vi "SimpleGit_Item_OnUpdateCommand.vi"(10 "Menu Item In":T1={"Menu Name"="", "Description"="", "Icon File Name"=path "", "Menu Tag"="", "Enabled"=TRUE, "Checked"=FALSE, "Separator"=FALSE, "Batchable"=TRUE, "Weight"=0, "Batch Mode (Ignored if Not Batchable)"=enum."Show If All Items Support Command", "Menu Location"=enum."<None>", "Exclude From Getting Started Window Menu"=FALSE}, 11 "Object":T2) -> (3 "Menu Item Out":T1={"Menu Name"="", "Description"="", "Icon File Name"=path "", "Menu Tag"="", "Enabled"=TRUE, "Checked"=FALSE, "Separator"=FALSE, "Batchable"=TRUE, "Weight"=0, "Batch Mode (Ignored if Not Batchable)"=enum."Show If All Items Support Command", "Menu Location"=enum."<None>", "Exclude From Getting Started Window Menu"=FALSE})   [LabVIEW 2017]
uses:
  <resource>/Framework/Providers/API/ItemRef.ctl
  <resource>/Framework/Providers/API/mxLvMenuItem.ctl
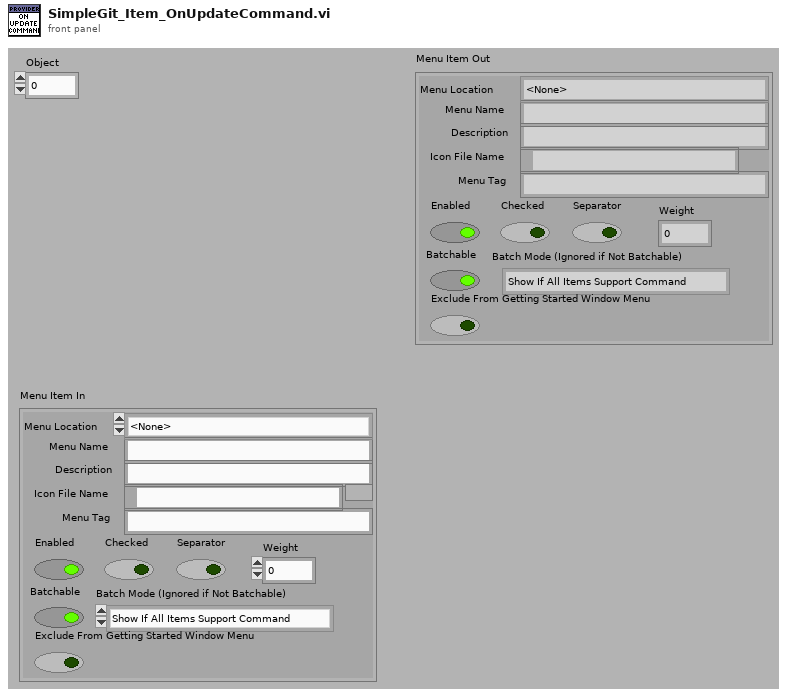
[diagram p1: front panel]
types:
  T1 = typedef "mxLvMenuItem.ctl" = cluster{"Menu Name":string, "Description":string, "Icon File Name":path, "Menu Tag":string, "Enabled":bool, "Checked":bool, "Separator":bool, "Batchable":bool, "Weight":i32, "Batch Mode (Ignored if Not Batchable)":enum32{"Show If All Items Support Command", "Show If Any Items Support Command"}, "Menu Location":enum32{"<None>", "Project", "Project / Build Specifications", "Tools", "Tools / Source Control", "Tools / Real-Time Module", "Help"}, "Exclude From Getting Started Window Menu":bool}
  T2 = typedef "ItemRef.ctl" = u64
  T3 = cluster{"current branch":string, "current commit":string, "Commit Info":string}
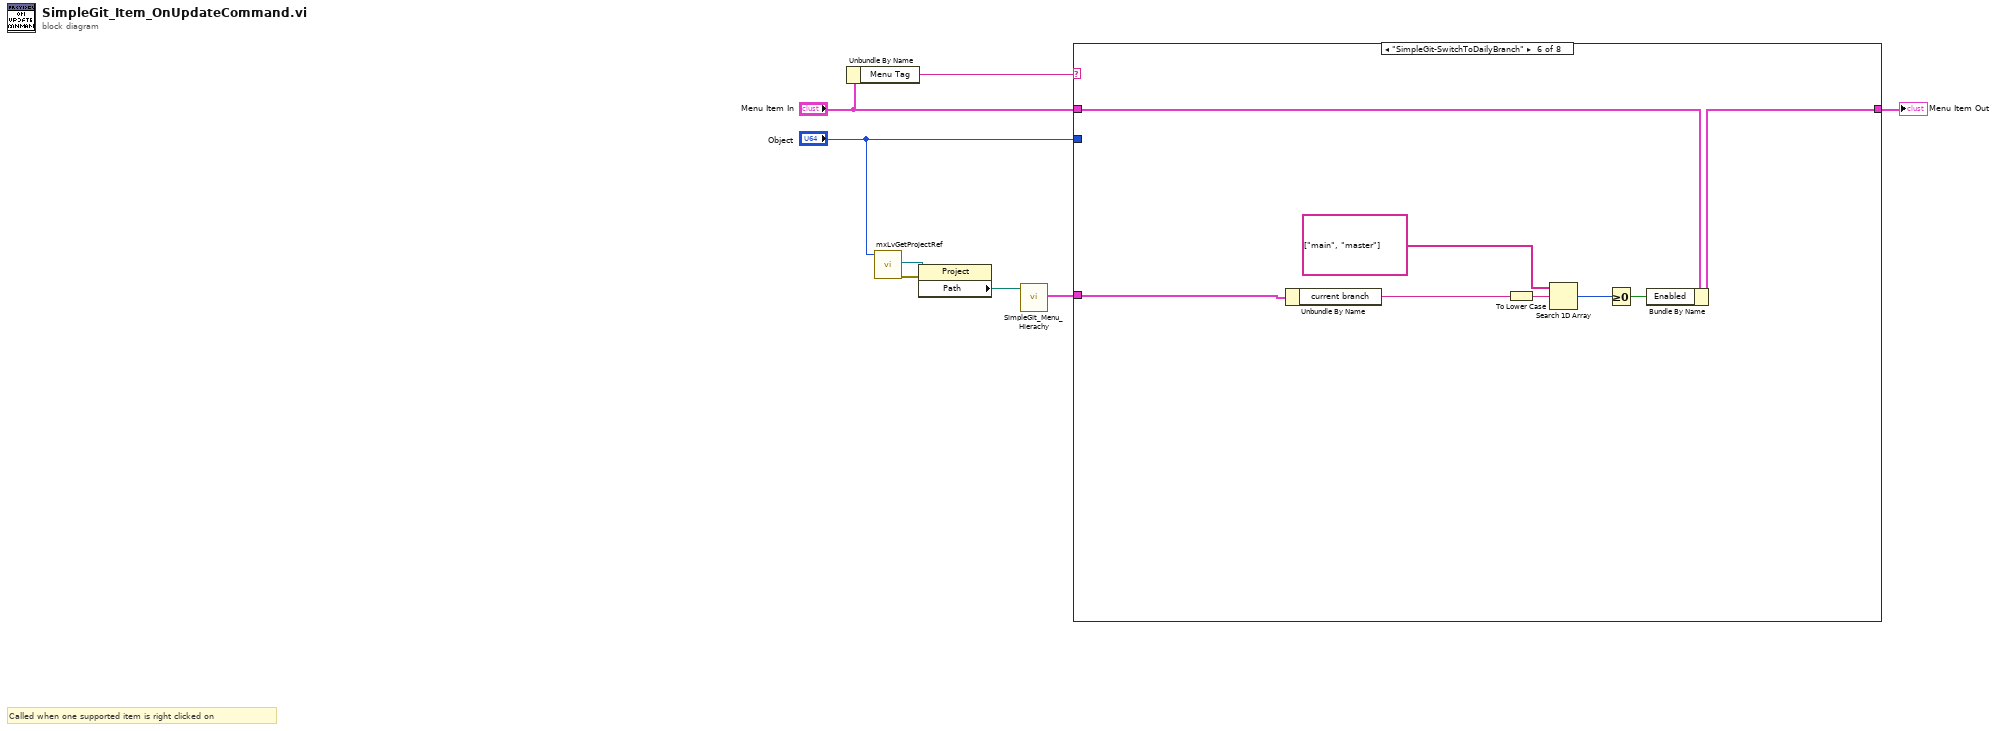
[diagram p0: block diagram]
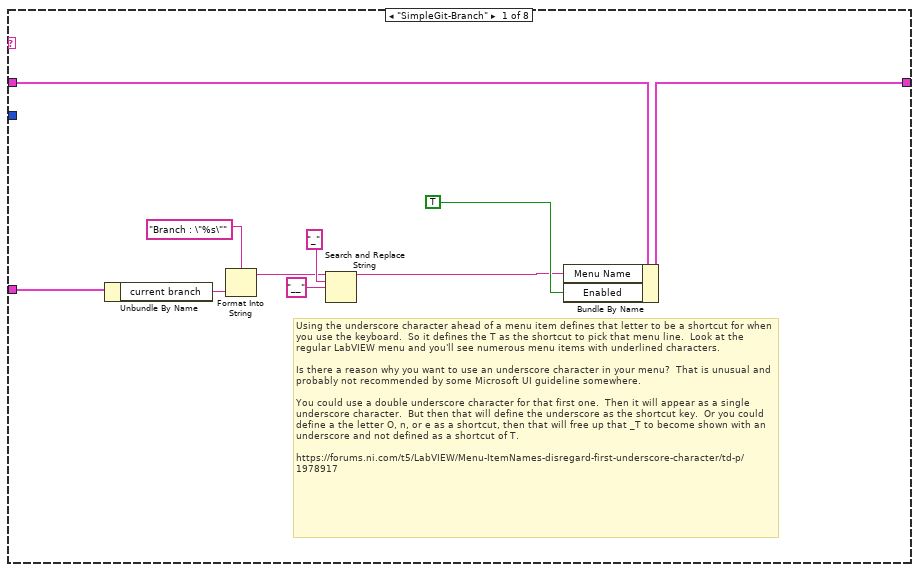
[diagram p2: hidden frame]
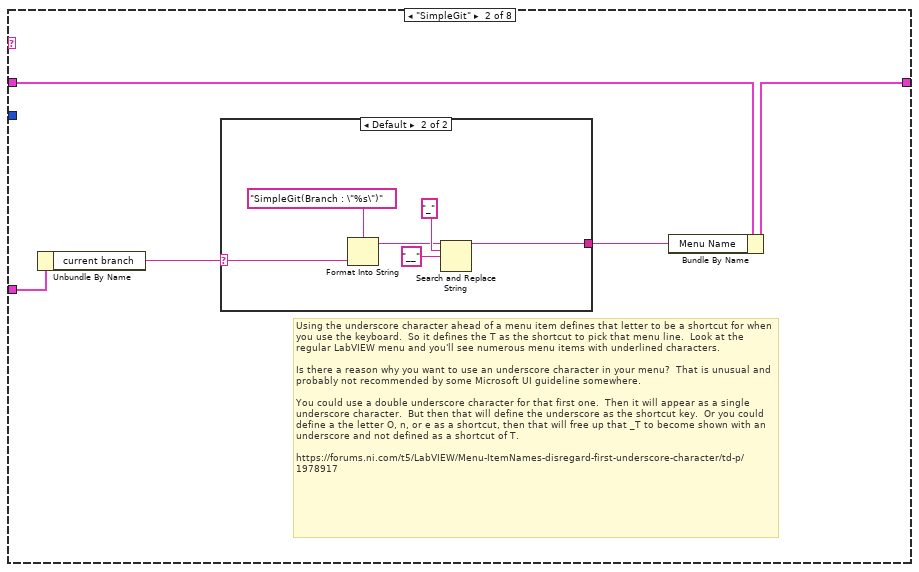
[diagram p3: hidden frame]
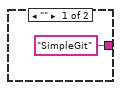
[diagram p4: hidden frame]
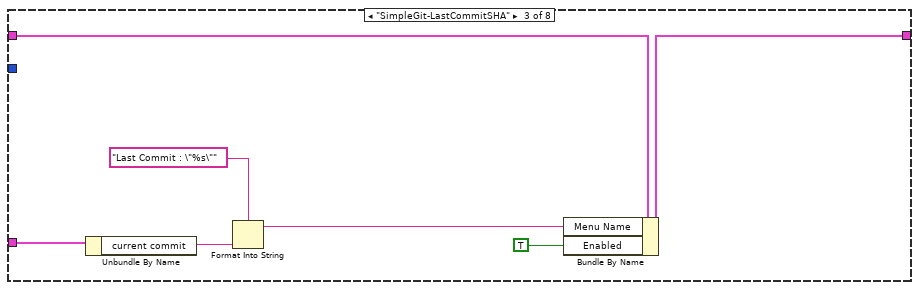
[diagram p5: hidden frame]
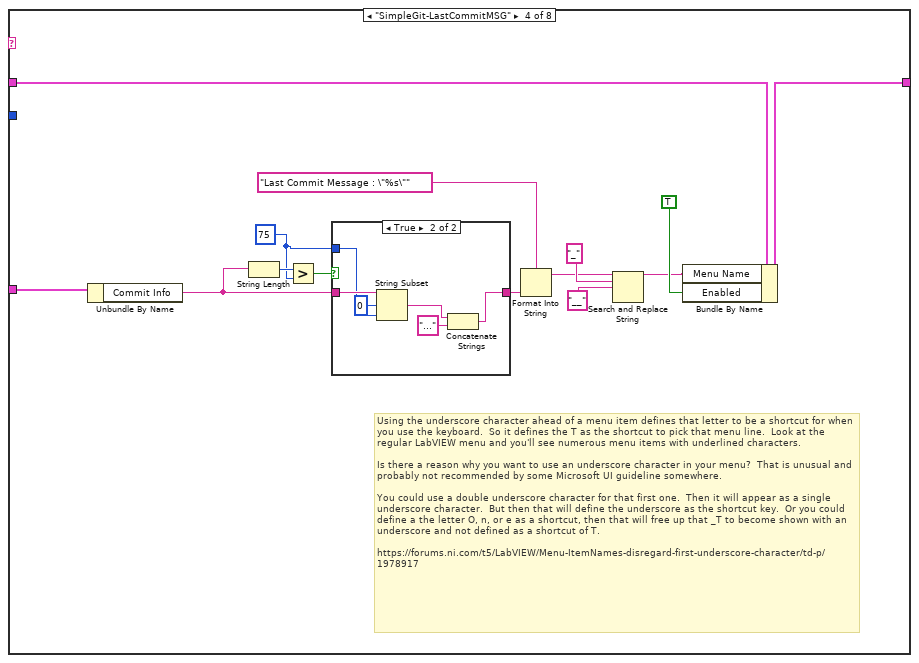
[diagram p6: hidden frame]
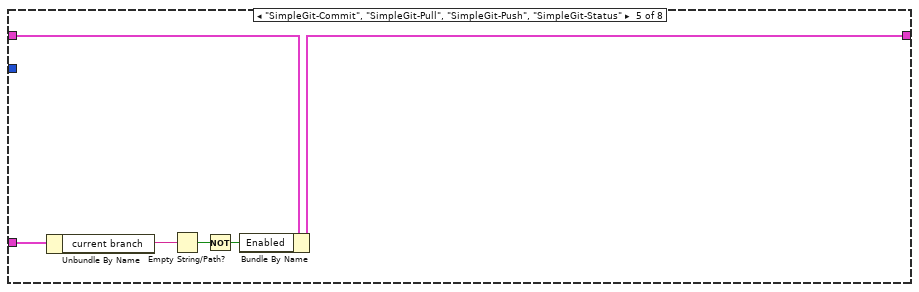
[diagram p8: hidden frame]
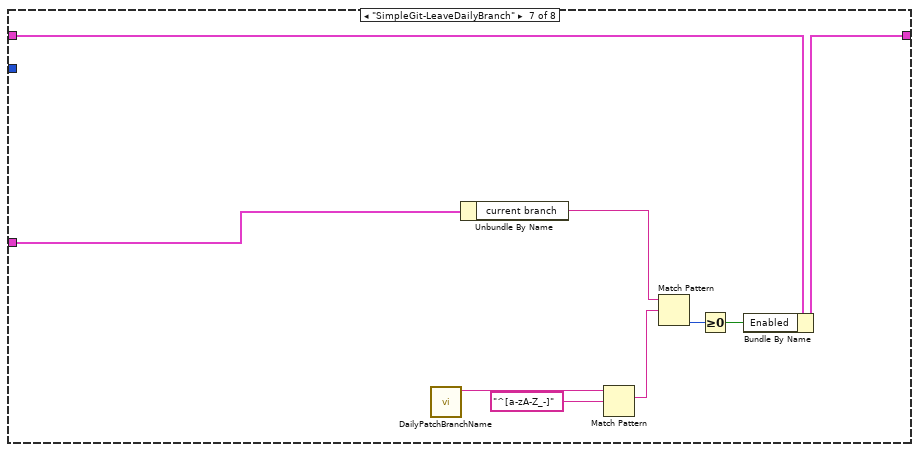
[diagram p9: hidden frame]
diagram:
  # "Called when one supported item is right clicked on"
  n1 = Unbundle By Name("Menu Item In") -> ("Menu Tag"=w8:string)
  n2 = call <resource>:"mxLvGetProjectRef.vi"("Item"="Object") -> ("error out"=w3:errorcluster, "Project Refnum"=w4:refnum<vi>)  [unwired: 8 in, 1 out]
  n3 = property class="Project"(reference=w4, error in=w3) -> ("Path"=w2:path)  [unwired: 2 out]
  n4 = call "SimpleGit_Menu_Hierachy.vi"("ProjectPath"=w2) -> ("branch info"=w1:T3)  [unwired: 9 in, 1 out]
  n5 = case shown="\"SimpleGit-SwitchToDailyBranch\"" w8 {
    tunnel: [w17 w22 w36 w50 w63 w71 w80 w82] -> w7
    tunnel: "Menu Item In" -> [w18 w23 w37 w51 w64 w72 w81 w82]
    tunnel: "Object" -> [_ _ _ _ _ _ _ _]
    tunnel: w1 -> [w9 w19 w32 w43 w60 w70 w74 _]
    frame "SimpleGit-Branch" {
      # "Using the underscore character ahead of a menu item defines that letter to be a shortcut for when you use the keyboard.  So it defines the T as the shortcut to pick that menu line.  Look at the regular LabVIEW menu and you'll see numerous menu items with underlined characters. \n\nIs there a reason why you want to use an underscore character in your menu?  That is unusual and probably not recommended by some Microsoft UI guideline somewhere.\n\nYou could use a double underscore character for that first one.  Then it will appear as a single underscore character.  But then that will define the underscore as the shortcut key.  Or you could define a the letter O, n, or e as a shortcut, then that will free up that _T to become shown with an underscore and not defined as a shortcut of T.\n\nhttps://forums.ni.com/t5/LabVIEW/Menu-ItemNames-disregard-first-underscore-character/td-p/1978917"
      n6 = Unbundle By Name(w9) -> ("current branch"=w10:string)
      n7 = Format Into String(format string="Branch : \"%s\"" ("string"), w10) -> (resulting string=w11:string)  [unwired: 2 in, 1 out]
      n8 = Search and Replace String(input string=w11, search string="_", replace string="__" ("replace string (\"\")")) -> (result string=w14:string)  [unwired: 5 in, 3 out]
      n9 = Bundle By Name(cluster=w18, "Menu Name"=w14, "Enabled"=TRUE) -> (w17:T1)
    }
    frame "SimpleGit" {
      # "Using the underscore character ahead of a menu item defines that letter to be a shortcut for when you use the keyboard.  So it defines the T as the shortcut to pick that menu line.  Look at the regular LabVIEW menu and you'll see numerous menu items with underlined characters. \n\nIs there a reason why you want to use an underscore character in your menu?  That is unusual and probably not recommended by some Microsoft UI guideline somewhere.\n\nYou could use a double underscore character for that first one.  Then it will appear as a single underscore character.  But then that will define the underscore as the shortcut key.  Or you could define a the letter O, n, or e as a shortcut, then that will free up that _T to become shown with an underscore and not defined as a shortcut of T.\n\nhttps://forums.ni.com/t5/LabVIEW/Menu-ItemNames-disregard-first-underscore-character/td-p/1978917"
      n10 = Unbundle By Name(w19) -> ("current branch"=w20:string)
      n11 = case shown="Default" w20 {
        selector: w20 -> [_ w25]
        tunnel: ["SimpleGit" ("result string") w29] -> w21
        frame "" {
        }
        frame Default {
          n12 = Format Into String(format string="SimpleGit(Branch : \"%s\")" ("string"), w25) -> (resulting string=w26:string)  [unwired: 2 in, 1 out]
          n13 = Search and Replace String(input string=w26, search string="_", replace string="__" ("replace string (\"\")")) -> (result string=w29:string)  [unwired: 5 in, 3 out]
        }
      }
      n14 = Bundle By Name(cluster=w23, "Menu Name"=w21) -> (w22:T1)
    }
    frame "SimpleGit-LastCommitSHA" {
      n15 = Unbundle By Name(w32) -> ("current commit"=w31:string)
      n16 = Format Into String(format string="Last Commit : \"%s\"" ("string"), w31) -> (resulting string=w33:string)  [unwired: 2 in, 1 out]
      n17 = Bundle By Name(cluster=w37, "Menu Name"=w33, "Enabled"=TRUE) -> (w36:T1)
    }
    frame "SimpleGit-LastCommitMSG" {
      w38 = 75 ("y")
      # "Using the underscore character ahead of a menu item defines that letter to be a shortcut for when you use the keyboard.  So it defines the T as the shortcut to pick that menu line.  Look at the regular LabVIEW menu and you'll see numerous menu items with underlined characters. \n\nIs there a reason why you want to use an underscore character in your menu?  That is unusual and probably not recommended by some Microsoft UI guideline somewhere.\n\nYou could use a double underscore character for that first one.  Then it will appear as a single underscore character.  But then that will define the underscore as the shortcut key.  Or you could define a the letter O, n, or e as a shortcut, then that will free up that _T to become shown with an underscore and not defined as a shortcut of T.\n\nhttps://forums.ni.com/t5/LabVIEW/Menu-ItemNames-disregard-first-underscore-character/td-p/1978917"
      n18 = Unbundle By Name(w43) -> ("Commit Info"=w42:string)
      n19 = String Length(string=w42) -> (length=w41:i32)
      n20 = Greater?(x=w41, y=w38) -> (0:w40:bool)
      n21 = case shown="True" w40 {
        tunnel: [w52 w53] -> w39
        tunnel: w42 -> [w52 w58]
        tunnel: w38 -> [_ w57]
        frame False {
        }
        frame True {
          n22 = String Subset(string=w58, offset (0)=0, length (rest)=w57) -> (substring=w55:string)
          n23 = Concatenate Strings(w55, "..." ("string")) -> (w53:string)
        }
      }
      n24 = Format Into String(format string="Last Commit Message : \"%s\"" ("string"), w39) -> (resulting string=w44:string)  [unwired: 2 in, 1 out]
      n25 = Search and Replace String(input string=w44, search string="_", replace string="__" ("replace string (\"\")")) -> (result string=w47:string)  [unwired: 5 in, 3 out]
      n26 = Bundle By Name(cluster=w51, "Menu Name"=w47, "Enabled"=TRUE) -> (w50:T1)
    }
    frame "SimpleGit-Commit", "SimpleGit-Pull", "SimpleGit-Push", "SimpleGit-Status" {
      n27 = Unbundle By Name(w60) -> ("current branch"=w59:string)
      n28 = Empty String/Path?(string/path=w59) -> (empty?=w62:bool)
      n29 = Not(x=w62) -> (.not. x?=w61:bool)
      n30 = Bundle By Name(cluster=w64, "Enabled"=w61) -> (w63:T1)
    }
    frame "SimpleGit-SwitchToDailyBranch" {
      n31 = Unbundle By Name(w70) -> ("current branch"=w69:string)
      n32 = To Lower Case(string=w69) -> (all lower case string=w68:string)
      n33 = Search 1D Array(1D array=string[] ["main", "master"] ("x"), element=w68) -> (index of element=w66:i32)  [unwired: 1 in]
      n34 = Greater Or Equal To 0?(x=w66) -> (x >= 0?=w65:bool)
      n35 = Bundle By Name(cluster=w72, "Enabled"=w65) -> (w71:T1)
    }
    frame "SimpleGit-LeaveDailyBranch" {
      n36 = call "DailyPatchBranchName.vi"() -> ("DailyPatchBranchName"=w77:string)  [unwired: 11 in]
      n37 = Unbundle By Name(w74) -> ("current branch"=w73:string)
      n38 = Match Pattern(string=w77, regular expression="^[a-zA-Z_-]") -> (match substring=w75:string)  [unwired: 1 in, 3 out]
      n39 = Match Pattern(string=w73, regular expression=w75) -> (offset past match=w79:i32)  [unwired: 1 in, 3 out]
      n40 = Greater Or Equal To 0?(x=w79) -> (x >= 0?=w78:bool)
      n41 = Bundle By Name(cluster=w81, "Enabled"=w78) -> (w80:T1)
    }
    frame Default {
    }
  }
  "Menu Item Out" <- w7
